vi "Grab from metadata.vi"(11 "Metadata in":string[][](array[string])) -> (1 "hours":dbl, 2 "sample":dbl, 3 "model":dbl)   [LabVIEW 2013]
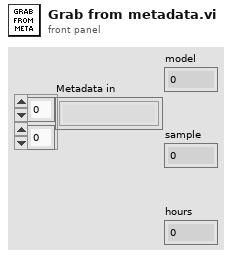
[diagram p1: front panel]
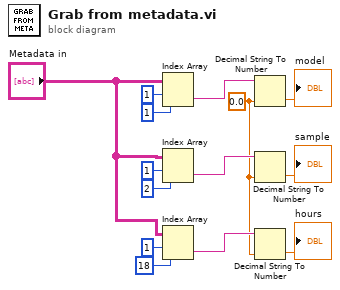
[diagram p0: block diagram]
diagram:
  w1 = 0.0 ("default (0 I32)")
  n1 = Index Array(array="Metadata in", index (row)=1, index (col)=1 ("disabled index (col)")) -> (element=w12:string)
  n2 = Index Array(array="Metadata in", index (row)=1, index (col)=2 ("disabled index (col)")) -> (element=w9:string)
  n3 = Index Array(array="Metadata in", index (row)=1, index (col)=18 ("disabled index (col)")) -> (element=w4:string)
  n4 = Decimal String To Number(string=w12, default (0L)=w1) -> (number=→"model":dbl)  [unwired: 1 in, 1 out]
  n5 = Decimal String To Number(string=w9, default (0L)=w1) -> (number=→"sample":dbl)  [unwired: 1 in, 1 out]
  n6 = Decimal String To Number(string=w4, default (0L)=w1) -> (number=→"hours":dbl)  [unwired: 1 in, 1 out]
